vi "HumanGetReverse.vi"() -> (3 "Reverse":bool)   [LabVIEW 2023]
uses:
  HumanGlobal.vi
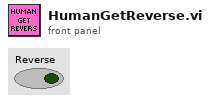
[diagram p1: front panel]
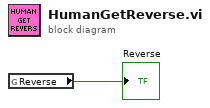
[diagram p0: block diagram]
diagram:
  n1 = global read "HumanGlobal.vi" "Reverse"() -> (→"Reverse":bool)
